vi "AbsolutePosition_KCubeInertial.vi"(9 "go to?":bool, 10 "set absolute position":i32, 11 ".NET Refnum in":refnum<k24>) -> ()   [LabVIEW 2019]
doc: "Set and run absolute position for KCube Inertial motors."
uses:
  D:/Victor Sun/optical trap control/Kinesis/Thorlabs.MotionControl.KCube.InertialMotorCLI.dll
  Kinesis/Thorlabs.MotionControl.KCube.InertialMotorCLI.dll
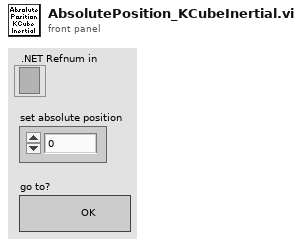
[diagram p1: front panel]
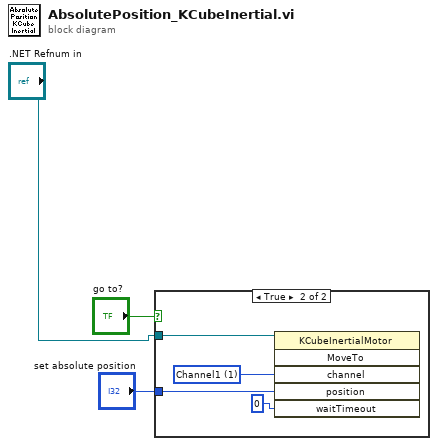
[diagram p0: block diagram]
diagram:
  n1 = case shown="True" "go to?" {
    tunnel: ".NET Refnum in" -> [_ w5]
    tunnel: "set absolute position" -> [_ w4]
    frame False {
    }
    frame True {
      w7 = 1 items=["Channel1"=1, "Channel2"=2, "Channel3"=3, "Channel4"=4] ("channel")
      n2 = invoke class="KCubeInertialMotor" method="MoveTo"(reference=w5, "channel"=w7, "position"=w4, "waitTimeout"=0) -> ()  [unwired: 2 in, 6 out]
    }
  }
